vi "Stop Resource.vi"(11 "Actor in":refnum<class "RefNums and UICtrl.lvclass">) -> (3 "Actor out":refnum<class "RefNums and UICtrl.lvclass">)   [LabVIEW 2020, in "RefNums and UICtrl.lvclass"]
uses:
  RefNums and UICtrl.lvclass
  RefNums and UICtrl.lvclass/RefNums and UICtrl.ctl
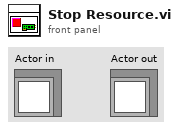
[diagram p1: front panel]
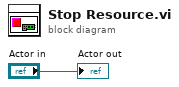
[diagram p0: block diagram]
diagram:
  "Actor out" <- "Actor in"
